vi "MAIN.vi"() -> ()   [LabVIEW 2022 SP3]
panel:
  in  "Button":bool
  in  "Results":string[][](table)
  in  "Key words to find:":string
  in  "Project Path":path
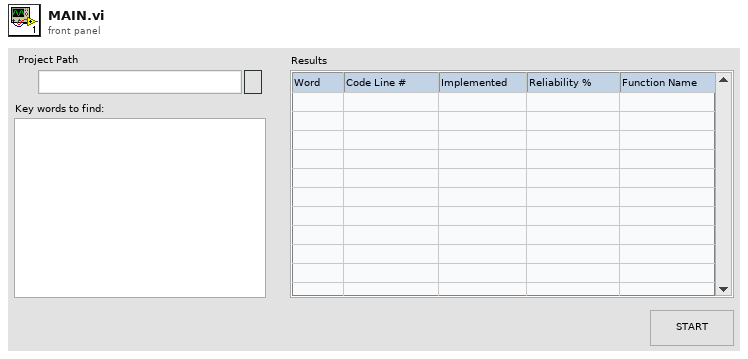
[diagram p1: front panel]
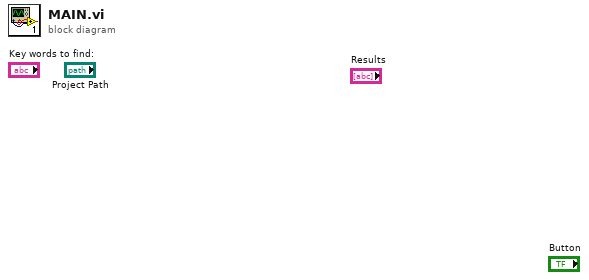
[diagram p0: block diagram]
diagram:
